vi "Read Value.vi"(8 "error in (no error)":errorcluster, 11 "Set Double Float in":refnum<class "Set Double Float.lvclass">) -> (0 "error out":errorcluster, 2 "Value":dbl, 3 "Set Double Float out":refnum<class "Set Double Float.lvclass">)   [LabVIEW 2021, in "BT.lvlib" / "Set Double Float.lvclass"]
uses:
  Set Double Float.lvclass
  Set Double Float.lvclass/Set Double Float.ctl
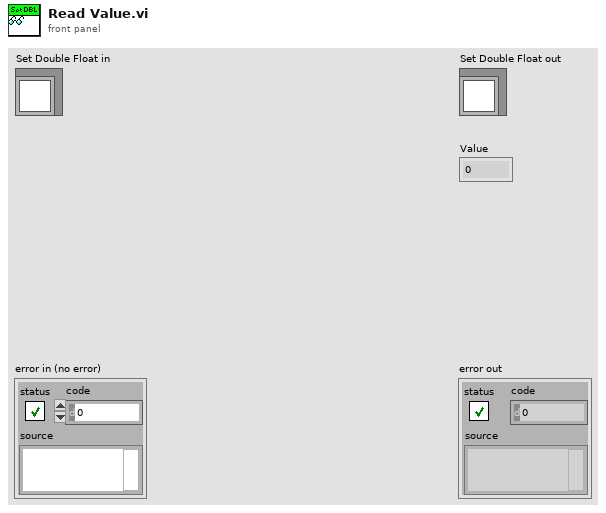
[diagram p1: front panel]
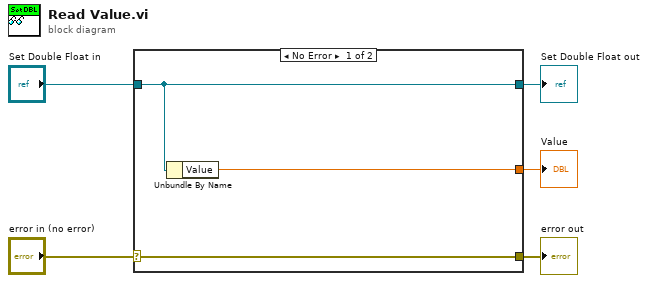
[diagram p0: block diagram]
diagram:
  n1 = case shown="No Error" "error in (no error)" {
    selector: "error in (no error)" -> [w8 w9]
    tunnel: [w8 w9] -> w4
    tunnel: [w7 w10] -> w2
    tunnel: "Set Double Float in" -> [w7 w10]
    tunnel: [w6 _] -> w1
    frame No Error {
      n2 = Unbundle By Name(w7) -> ("Value"=w6:dbl)
    }
    frame Error {
    }
  }
  "error out" <- w4
  "Set Double Float out" <- w2
  "Value" <- w1
